vi "URAPICompile.vi"(2 "Script":string) -> (0 "trimmed script":string)   [LabVIEW 2014]
panel:
  out "Array":string[](array[string])
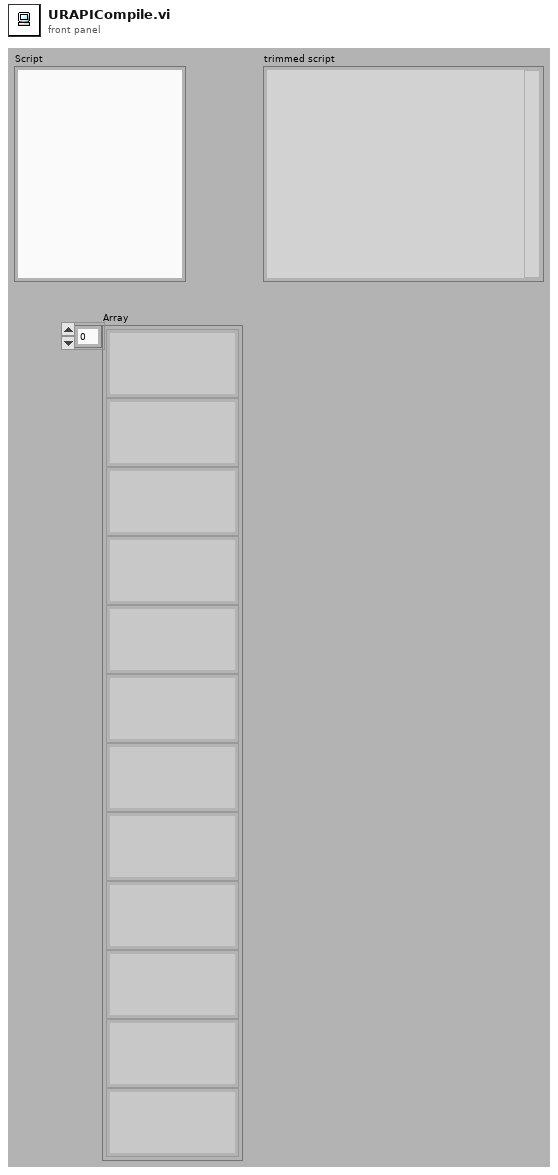
[diagram p1: front panel]
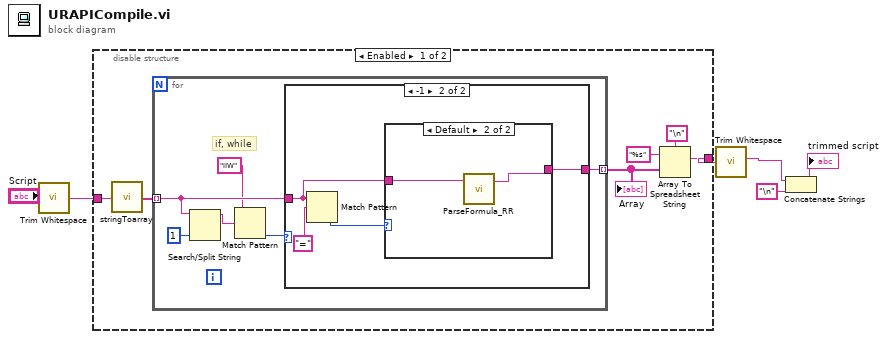
[diagram p0: block diagram]
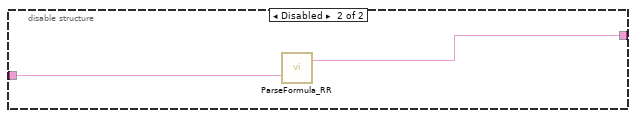
[diagram p4: hidden frame]
diagram:
  n1 = call <vilib>:"Trim Whitespace.vi"("string"="Script") -> ("trimmed string"=w2:string)  [unwired: 1 in]
  n2 = disable-structure shown="Enabled" {
    disable-tunnel: w2 -> [w8 w28]
    disable-tunnel: [w7 w27] -> w3
    frame Enabled {
      n3 = call <userlib>:"stringToarray.vi"("String"=w8) -> ("Array"=w11:string[])
      n4 = for {
        tunnel: w11 -> [w17] mode=indexing
        tunnel: [w18] -> w12 mode=indexing
        # "if, while"
        n5 = Search/Split String(string=w17, offset (0)=1) -> (substring before match=w15:string)  [unwired: 1 in, 2 out]
        n6 = Match Pattern(string="iIW" ("search string/char (-)"), regular expression=w15) -> (offset past match=w13:i32)  [unwired: 1 in, 3 out]
        n7 = case shown="-1" w13 {
          tunnel: [w19 w21] -> w18
          tunnel: w17 -> [w19 w20]
          frame 0, Default {
          }
          frame -1 {
            n8 = Match Pattern(string=w20, regular expression="=") -> (offset past match=w22:i32)  [unwired: 1 in, 3 out]
            n9 = case shown="Default" w22 {
              tunnel: [w24 w25] -> w21
              tunnel: w20 -> [w24 w26]
              frame -1 {
              }
              frame Default {
                n10 = call <userlib>:"ParseFormula_RR.vi"("Script"=w26) -> ("URAPI"=w25:string)  [unwired: 2 in]
              }
            }
          }
        }
      }
      "Array" <- w12
      n11 = Array To Spreadsheet String(delimiter (Tab)="\n", array=w12, 3:"%s" ("format string")) -> (spreadsheet string=w7:string)
    }
    frame Disabled {
      n12 = call <userlib>:"ParseFormula_RR.vi"("Script"=w28) -> ("URAPI"=w27:string)  [unwired: 2 in]
    }
  }
  n13 = call <vilib>:"Trim Whitespace.vi"("string"=w3) -> ("trimmed string"=w1:string)  [unwired: 1 in]
  n14 = Concatenate Strings(w1, "\n" ("command")) -> (→"trimmed script":string)
